vi "Read Complex Extended 1D Value.vi"(8 "error in (no error)":errorcluster, 11 "Numeric in":refnum<class "Abs_Complex Extended Float 1D.lvclass">) -> (0 "error out":errorcluster, 2 "Complex Double Float":cxt[](array[numeric]), 3 "Numeric out":refnum<class "Abs_Complex Extended Float 1D.lvclass">)   [LabVIEW 2021, in "Abs_Complex Extended Float 1D.lvclass"]
uses:
  Abs_Complex Extended Float 1D.lvclass
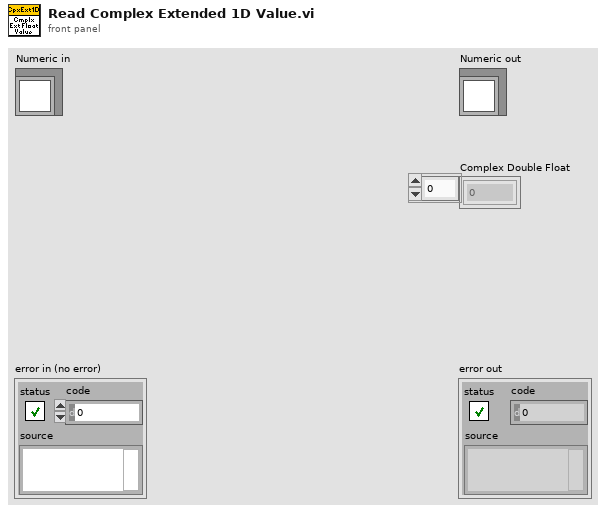
[diagram p1: front panel]
types:
  T1 = typedef "Abs_Complex Extended Float 1D.lvclass/Type.ctl" = cxt[]
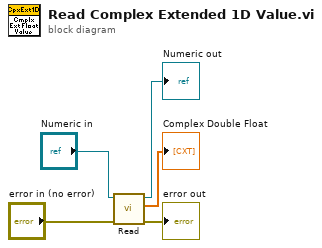
[diagram p0: block diagram]
diagram:
  n1 = call-dynamic "Read.vi"("error in (no error)"="error in (no error)", "Double Float.lvclass_340760 in"="Numeric in") -> ("error out"=→"error out":errorcluster, "Value"=→"Complex Double Float":T1, "Double Float.lvclass_340760 out"=→"Numeric out":refnum<class "Abs_Complex Extended Float 1D.lvclass">)  [unwired: 7 in]
